vi "查询-累积剂量记录.vi"() -> ()   [LabVIEW 2017]
uses:
  <vilib>/addons/database/Connection.llb/Conn ObjectReference.ctl
  <vilib>/Utility/inputDevices.llb/mouseAcquire.vi
  <vilib>/addons/database/NI_Database_API.lvlib
panel:
  out "信号-导出数据":bool=TRUE
  in  "停止？":bool=TRUE
  in  "提示-条件区域[]":string[](array[string])
  in  "提示-数据列表[]":string[](array[string])
  in  "提示-设备列表[]":string[](array[string])
  out "信号-重连DB":bool=TRUE
  in  "device ID":refnum<k1> caption="设备ID"
  out "信号-刷新功能管理表":bool=TRUE
  out "最小记录时间":i32[](array[numeric])
  out "DB 引用":T1
  out "累积功能管理":enum16{"设备列表"}(ring)
  out "提示-设备列表":string
  in  "全选-设备":bool
  in  "查询条件":T2
  in  "设备累积管理":i32[](listbox)
  out "累积剂量查询":enum16{"累积剂量查询"}(ring)
  out "提示-数据列表":string
  in  "记录类型":enum16{"全部记录", "报警记录"}(ring)
  in  "全选-记录":bool
  in  "记录列表":i32[](listbox)
  out "查询条件":enum16{"查询条件"}(ring)
  out "提示-条件区域":string
  out "查询状态":string
  out "选中状态":string
  out "起始时间":enum16{"起始时间"}(ring)
  in  "从今天":bool
  in  "起始年":u16(ring) items=["2017年"=2017]
  in  "起始月":u16(ring) items=["1月"=1, "2月"=2, "3月"=3, "4月"=4, "5月"=5, "6月"=6, "7月"=7, "8月"=8, "9月"=9, "10月"=10, "11月"=11, "12月"=12]
  in  "起始日":u16(ring) items=["1日"=1, "2日"=2, "3日"=3, "4日"=4, "5日"=5, "6日"=6, "7日"=7, "8日"=8, "9日"=9, "10日"=10, "11日"=11, "12日"=12, "13日"=13, "14日"=14, "15日"=15, "16日"=16, "17日"=17, "18日"=18, "19日"=19, "20日"=20, "21日"=21, "22日"=22, "23日"=23, "24日"=24, "25日"=25, "26日"=26, "27日"=27, "28日"=28, "29日"=29, "30日"=30, "31日"=31]
  out "截止时间":enum16{"截止时间"}(ring)
  in  "到今天":bool
  in  "截止年":u16(ring) items=["2017年"=2017]
  in  "截止月":u16(ring) items=["1月"=1, "2月"=2, "3月"=3, "4月"=4, "5月"=5, "6月"=6, "7月"=7, "8月"=8, "9月"=9, "10月"=10, "11月"=11, "12月"=12]
  in  "截止日":u16(ring) items=["1日"=1, "2日"=2, "3日"=3, "4日"=4, "5日"=5, "6日"=6, "7日"=7, "8日"=8, "9日"=9, "10日"=10, "11日"=11, "12日"=12, "13日"=13, "14日"=14, "15日"=15, "16日"=16, "17日"=17, "18日"=18, "19日"=19, "20日"=20, "21日"=21, "22日"=22, "23日"=23, "24日"=24, "25日"=25, "26日"=26, "27日"=27, "28日"=28, "29日"=29, "30日"=30, "31日"=31]
  in  "导出数据":bool
  in  "查询今日":bool
  in  "查看导出目录":bool
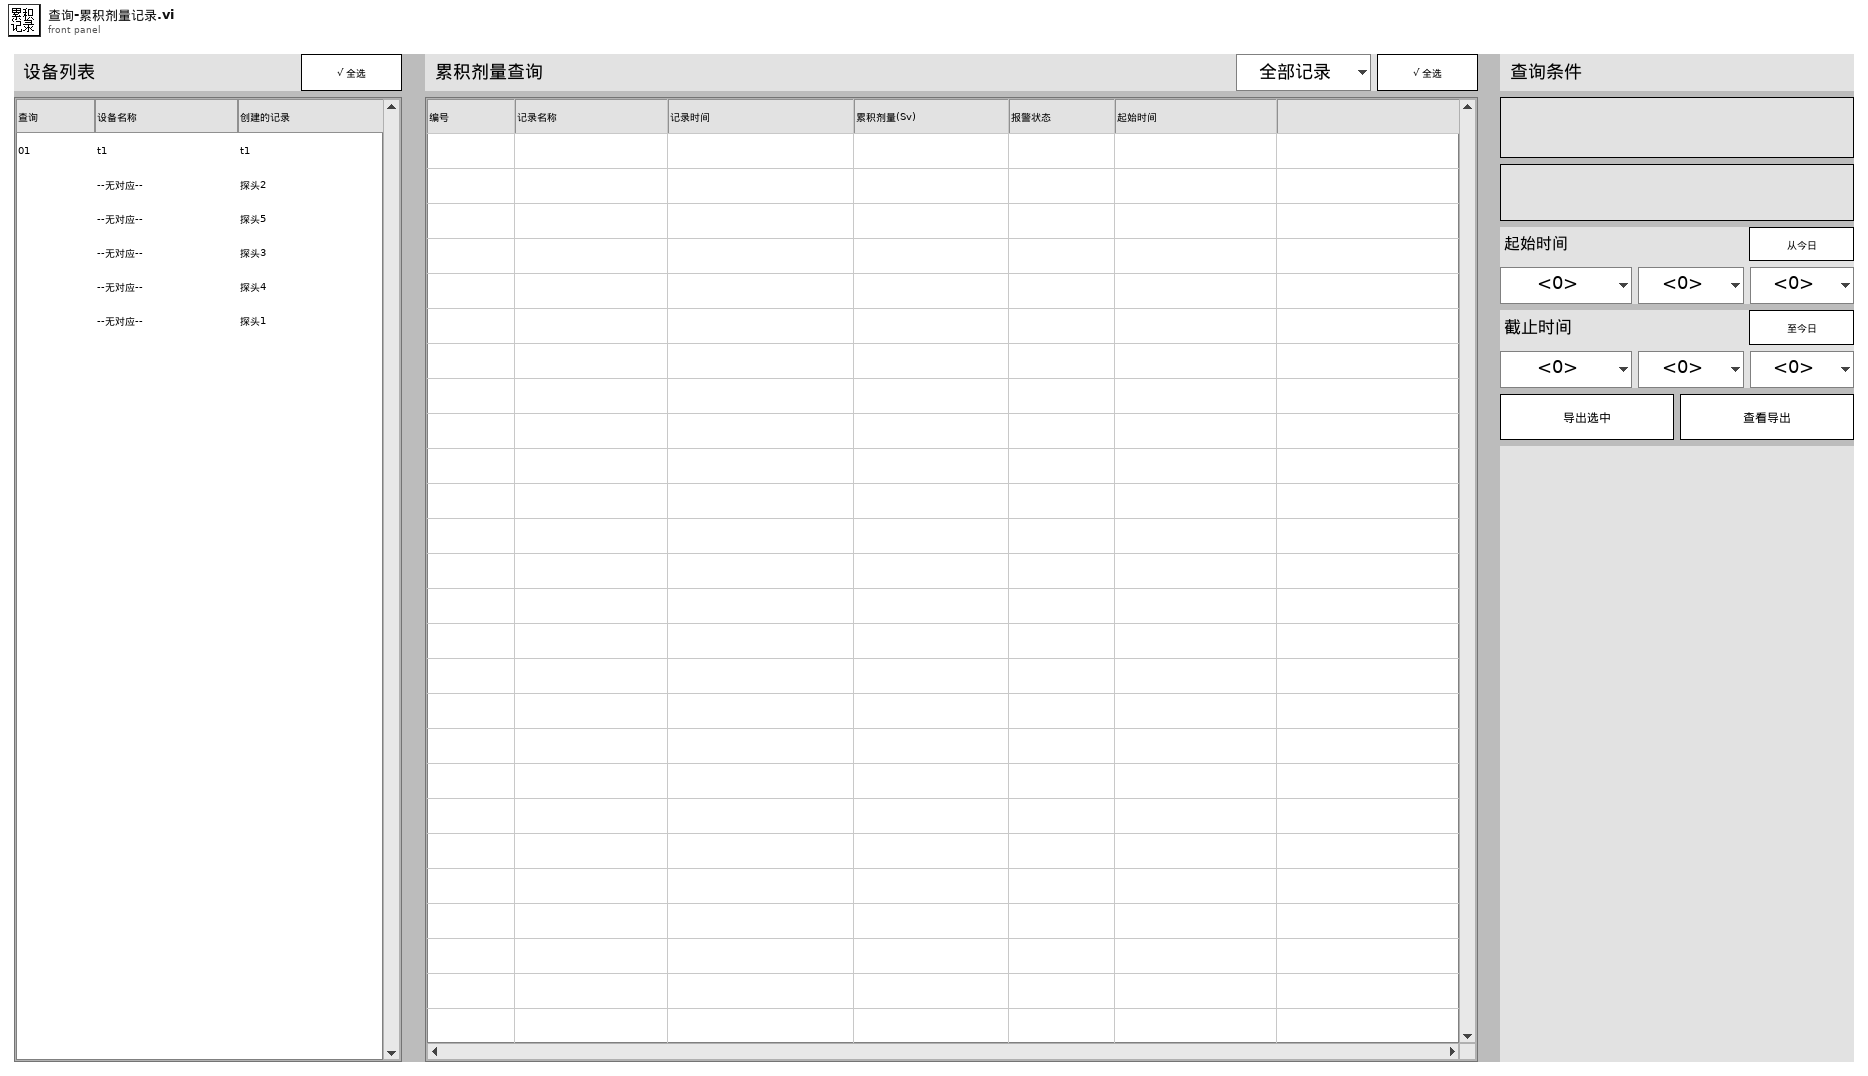
[diagram p1: front panel]
types:
  T1 = typedef "NI_Database_API.lvlib/Conn ObjectReference.ctl" = refnum<k1>
  T2 = cluster{"表名":string[], "起始时间":string, "截止时间":string, "优先排序":enum16{"表名优先", "记录时间优先"}, "排序方向":enum16{"升序", "降序"}, "记录类型":enum16{"全部记录", "报警记录"}}
  T3 = cluster{"设备名称":string, "启用累积？":bool, "起始时间":timestamp, "累积剂量":dbl, "累积报警阈值":dbl}
  T4 = typedef "LVDateTimeRec.ctl" = cluster{"秒数的小数部分":dbl, "秒":i32, "分":i32, "时":i32, "日":i32, "月":i32, "年":i32, "天数（周）":i32, "天数（年）":i32, "DST":i32}
  T5 = typedef "LVPoint32TypeDef.ctl" = cluster{"Horizontal":i32, "Vertical":i32}
  T6 = cluster{"button 1":bool, "button 2":bool, "button 3":bool, "button 4":bool}
  T7 = typedef "LVRowAndColumnTypeDef.ctl" = cluster{"Row":i32, "Column":i32}
  T8 = cluster{"设备名称":string, "启用累积？":bool, "起始时间":timestamp, "累积剂量":dbl, "累积报警阈值":dbl}[]
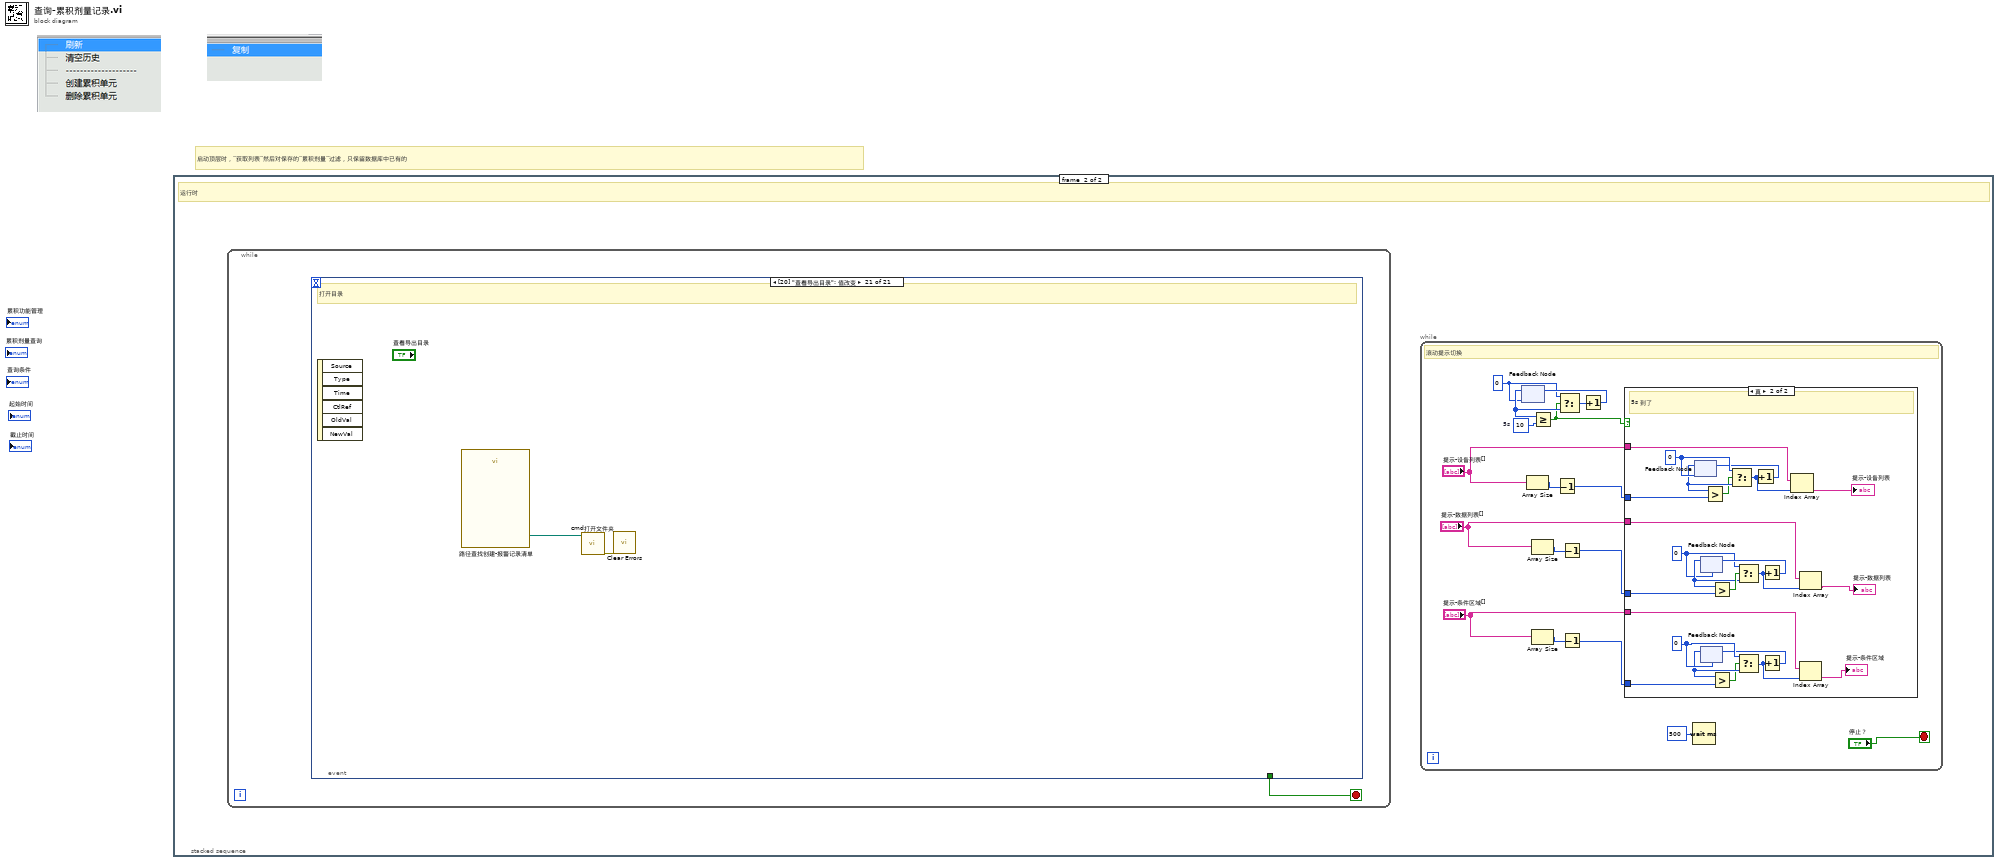
[diagram p0: block diagram]
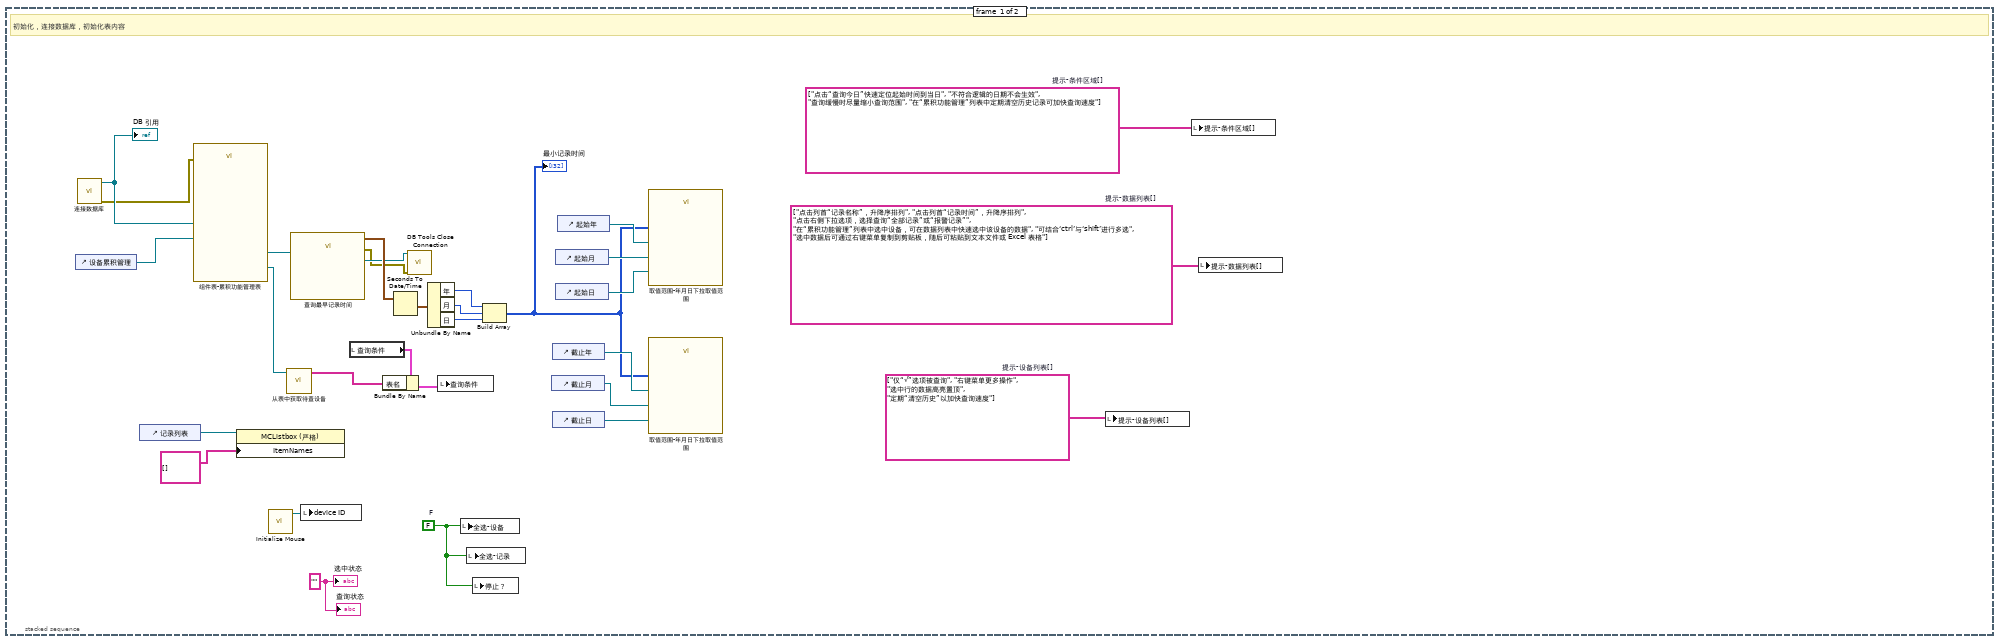
[diagram p2: hidden frame]
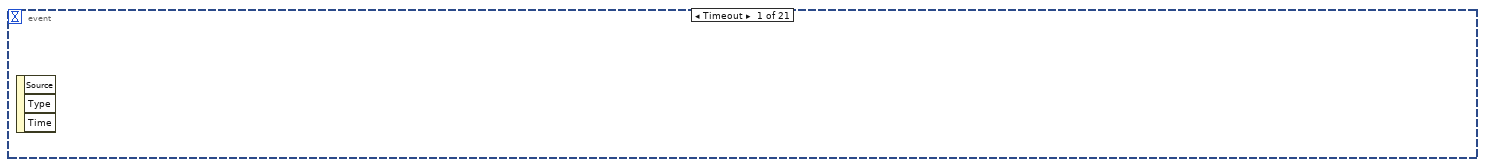
[diagram p4: hidden frame]
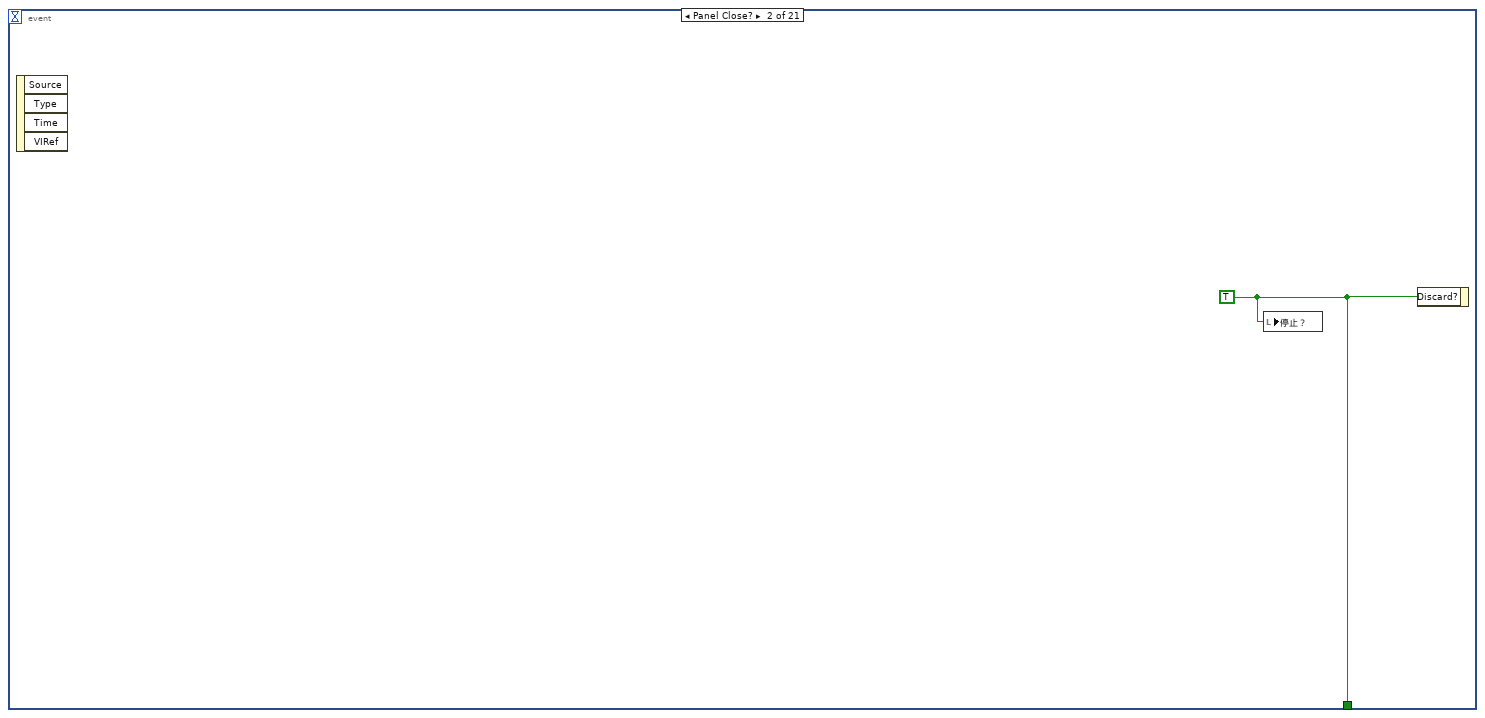
[diagram p5: hidden frame]
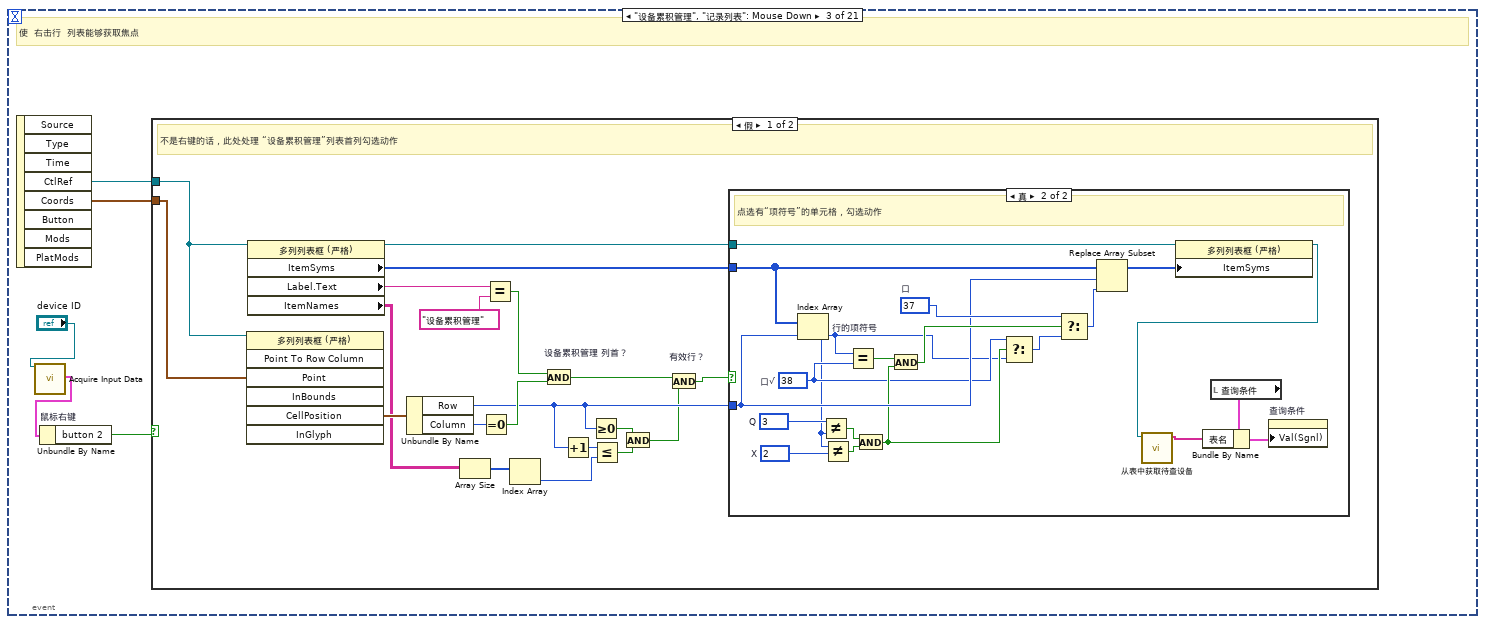
[diagram p6: hidden frame]
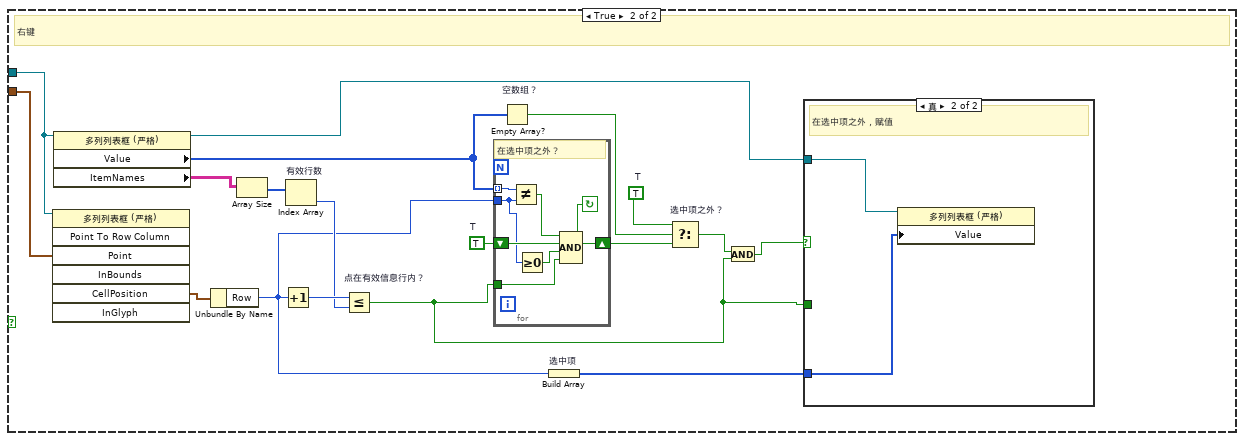
[diagram p8: hidden frame]
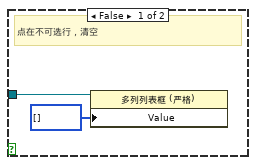
[diagram p10: hidden frame]
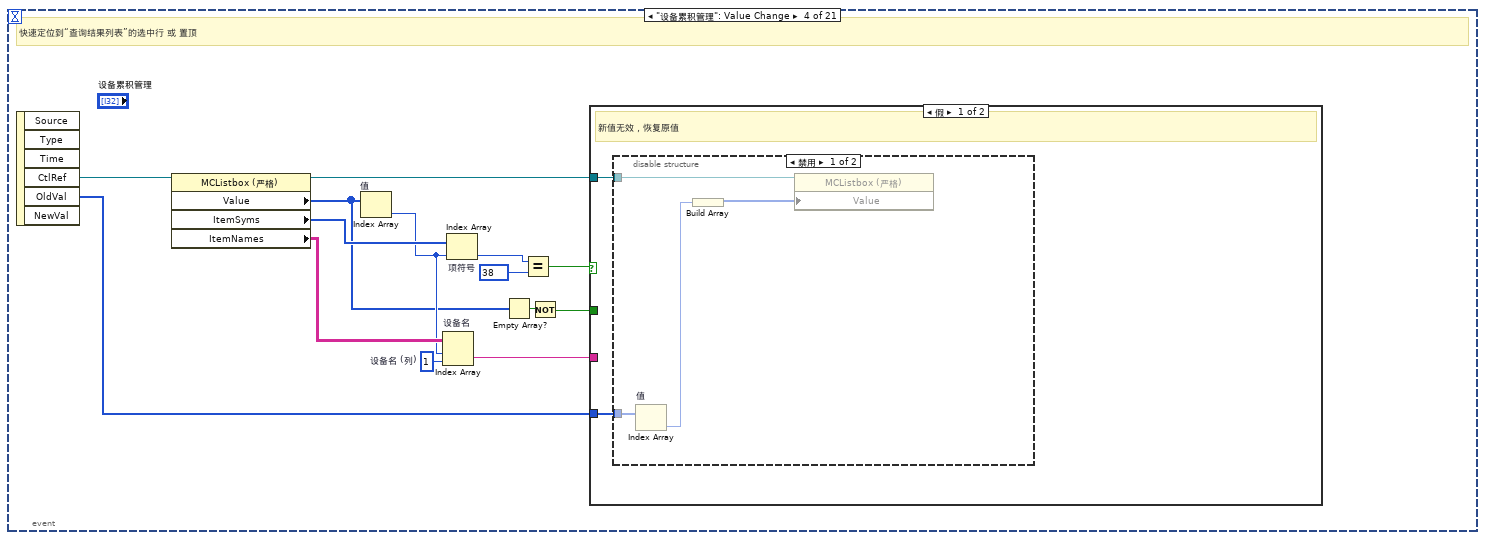
[diagram p11: hidden frame]
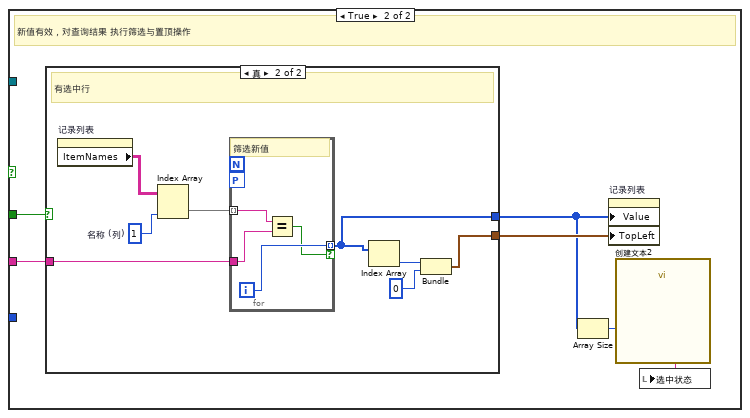
[diagram p13: hidden frame]
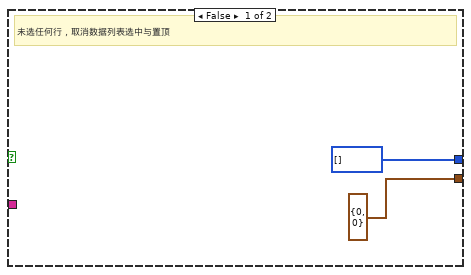
[diagram p14: hidden frame]
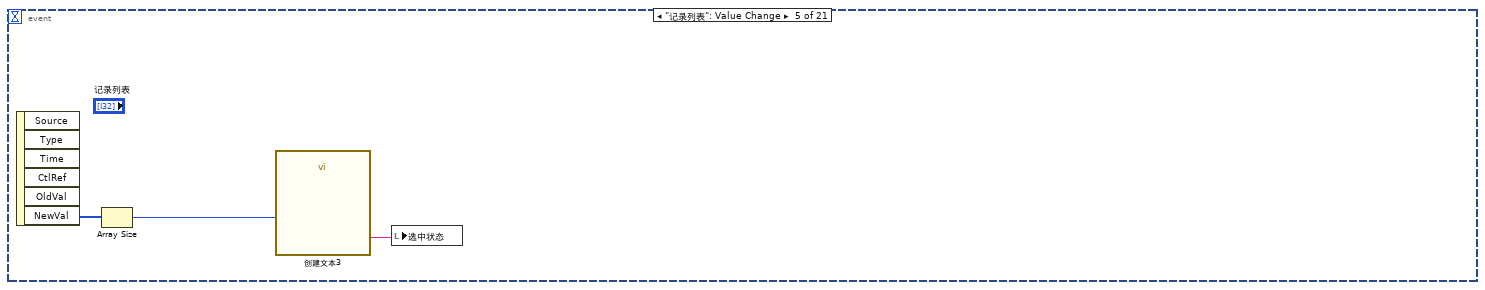
[diagram p15: hidden frame]
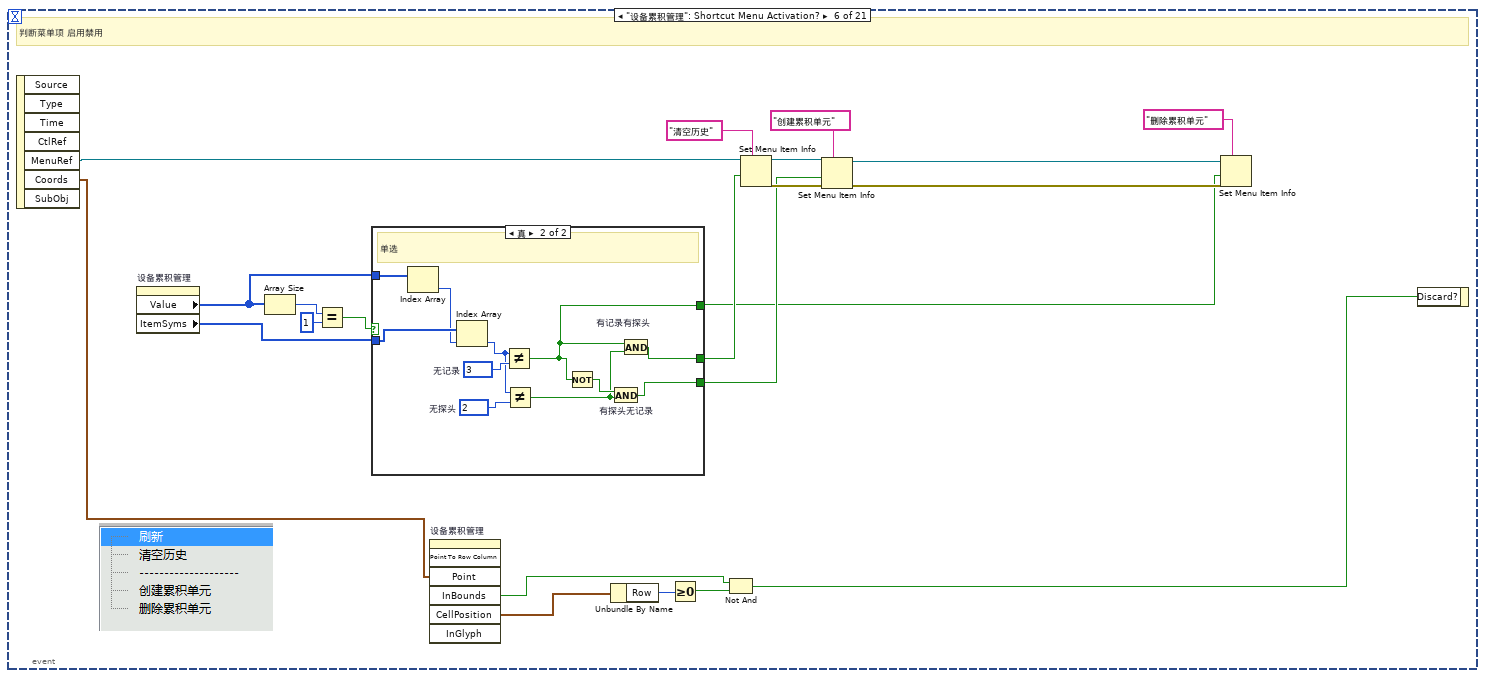
[diagram p16: hidden frame]
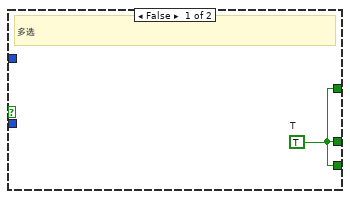
[diagram p17: hidden frame]
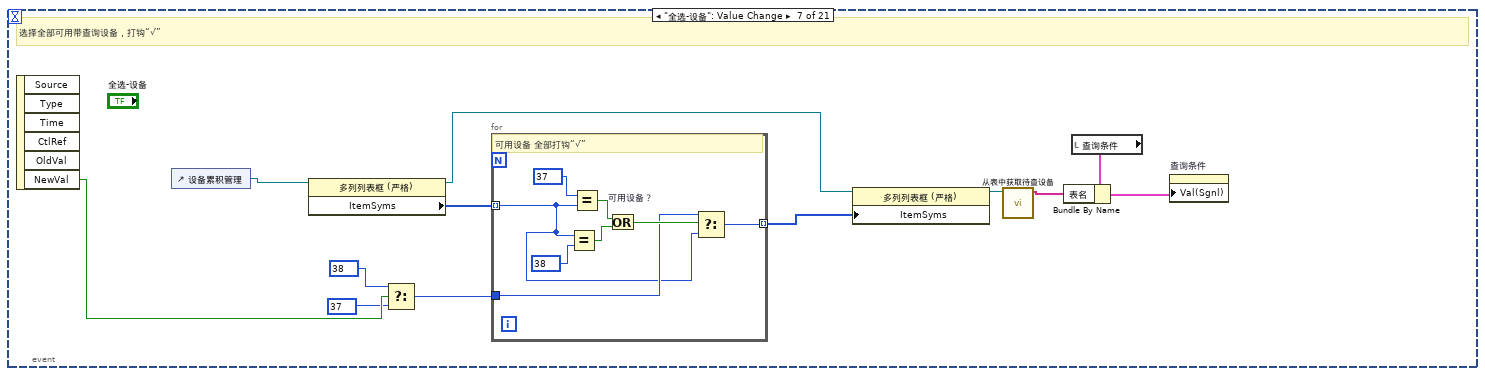
[diagram p18: hidden frame]
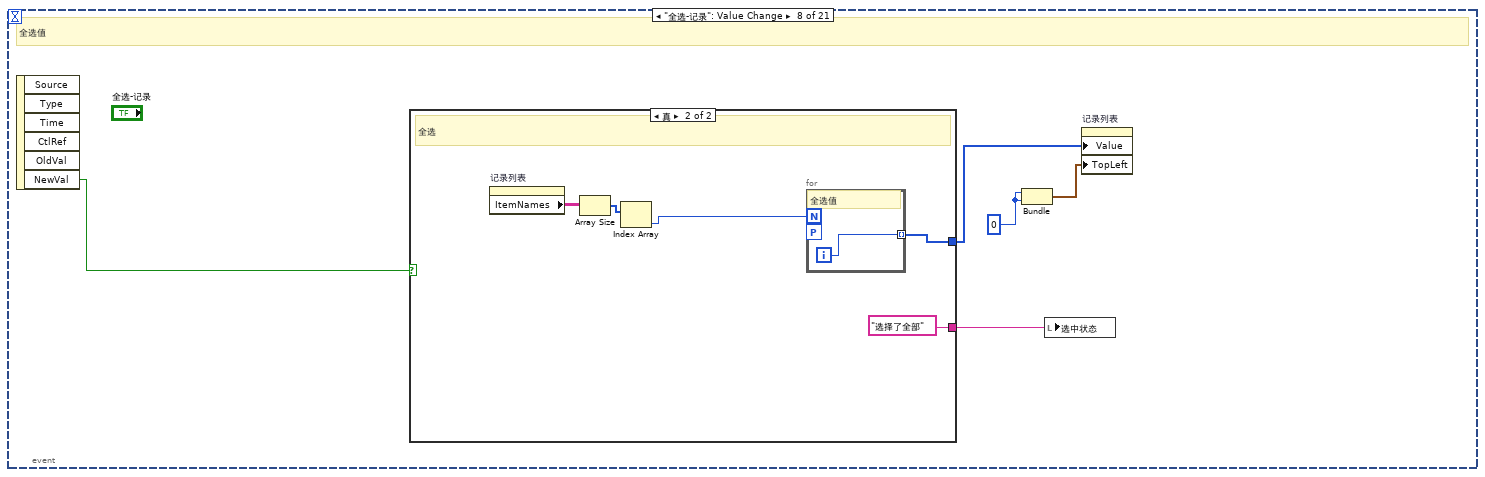
[diagram p19: hidden frame]
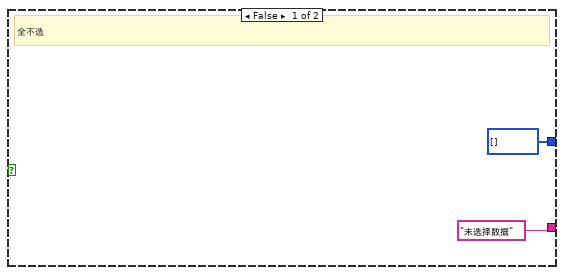
[diagram p20: hidden frame]
diagram:
  # "启动顶层时，“获取列表”然后对保存的“累积剂量”过滤，只保留数据库中已有的"
  n1 = stacked-sequence {
    frame #0 {
      w9 = string[] ["点击“查询今日”快速定位起始时间到当日", "不符合逻辑的日期不会生效", "查询缓慢时尽量缩小查询范围", "在“累积功能管理”列表中定期清空历史记录可加快查询速度"]  # 提示-条件区域[]
      w8 = string[] ["点击列首“记录名称”，升降序排列", "点击列首“记录时间”，升降序排列", "点击右侧下拉选项，选择查询“全部记录”或“报警记录”", "在“累积功能管理”列表中选中设备，可在数据列表中快速选中该设备的数据", "可结合‘ctrl’与‘shift’进行多选", "选中数据后可通过右键菜单复制到剪贴板，随后可粘贴到文本文件或 Excel 表格"]  # 提示-数据列表[]
      w10 = "" ("选中状态")
      w7 = string[] ["仅“√”选项被查询", "右键菜单更多操作", "选中行的数据高亮置顶", "定期“清空历史”以加快查询速度"]  # 提示-设备列表[]
      w6 = FALSE  # F
      # "初始化，连接数据库，初始化表内容"
      n2 = control-ref of="设备累积管理"() -> (w30:refnum<vi>)
      n3 = call "连接数据库.vi"() -> ("error out"=w3:errorcluster, "connection reference"=w16:T1)  [unwired: 10 in]
      "DB 引用" <- w16
      n4 = control-ref of="记录列表"() -> (w5:refnum<vi>)
      n5 = call "组件表-累积功能管理表.vi"("引用-累积功能管理列表"=w30, "error in (no error)"=w3, "DB 引用"=w16) -> ("数据库连接引用 o"=w29:T1, "引用-累积功能管理表 o"=w14:refnum<vi>)  [unwired: 6 in, 1 out]
      n6 = property class="MCListbox (严格)"(reference=w5, "ItemNames"=string[][] [] ("项名")) -> ()  [unwired: 1 in, 2 out]
      n7 = call <vilib>:"Initialize Mouse.vi"() -> ("device ID"=w15:refnum<k1>)  [unwired: 10 in, 1 out]
      n8 = call "从表中获取待查设备.vi"("引用-设备累积管理 i"=w14) -> ("选中的查询设备"=w12:string[])  [unwired: 10 in]
      n9 = call "查询最早记录时间.vi"("DB 引用"=w29) -> ("error out"=w1:errorcluster, "最小记录时间"=w22:timestamp, "数据库连接引用out"=w2:T1)  [unwired: 8 in]
      n10 = local write "device ID"(w15) -> ()
      n11 = local read "查询条件"() -> (w13:T2)
      n12 = Bundle By Name(cluster=w13, "表名"=w12) -> (w11:T2)
      n13 = Seconds To Date/Time(time stamp (now)=w22) -> (date time rec=w21:T4)  [unwired: 1 in]
      n14 = call <vilib>:"DB Tools Close Connection.vi"("error in (no error)"=w1, "connection reference"=w2) -> ()  [unwired: 5 in, 1 out]
      n15 = Unbundle By Name(w21) -> ("年"=w20:i32, "月"=w19:i32, "日"=w18:i32)
      n16 = local write "查询条件"(w11) -> ()
      n17 = local write "全选-设备"(w6) -> ()
      n18 = local write "全选-记录"(w6) -> ()
      n19 = local write "停止？"(w6) -> ()
      n20 = Build Array(w20, w19, w18) -> (w17:i32[])
      "最小记录时间" <- w17
      n21 = control-ref of="截止月"() -> (w24:refnum<vi>)
      n22 = control-ref of="截止年"() -> (w25:refnum<vi>)
      n23 = control-ref of="截止日"() -> (w23:refnum<vi>)
      n24 = control-ref of="起始月"() -> (w27:refnum<vi>)
      n25 = control-ref of="起始日"() -> (w26:refnum<vi>)
      n26 = control-ref of="起始年"() -> (w28:refnum<vi>)
      n27 = call "取值范围-年月日下拉取值范围.vi"("最小日期"=w17, "日"=w26, "月"=w27, "年"=w28) -> ()  [unwired: 7 in, 1 out]
      n28 = call "取值范围-年月日下拉取值范围.vi"("最小日期"=w17, "日"=w23, "月"=w24, "年"=w25) -> ()  [unwired: 7 in, 1 out]
      n29 = local write "提示-设备列表[]"(w7) -> ()
      n30 = local write "提示-条件区域[]"(w9) -> ()
      n31 = local write "提示-数据列表[]"(w8) -> ()
      "查询状态" <- w10
      "选中状态" <- w10
    }
    frame #1 {
      # "运行时"
      n32 = while {
        stop <- w72 stop-if-true
        n33 = event shown="[20] \"查看导出目录\": 值改变" {
          selector: _ -> [_ _ _ _ _ _ _ _ _ _ _ _ _ _ _ _ _ _ _ _ _]
          dyn-events: _ -> [_ _ _ _ _ _ _ _ _ _ _ _ _ _ _ _ _ _ _ _ _]
          timeout: _ -> [_ _ _ _ _ _ _ _ _ _ _ _ _ _ _ _ _ _ _ _ _]
          tunnel: [_ w73 _ _ _ _ _ _ _ _ _ _ _ _ _ _ _ _ _ _ _] -> w72
          event Timeout {
            n34 = event-data() -> ()  [unwired: 1 in, 3 out]
          }
          event Panel Close? {
            w73 = TRUE ("放弃？")
            n35 = event-data() -> ()  [unwired: 1 in, 4 out]
            n36 = local write "停止？"(w73) -> ()
            n37 = event-data("Discard?"=w73) -> ()  [unwired: 1 in, 1 out]
          }
          event "设备累积管理", "记录列表": Mouse Down {
            # "使  右击行  列表能够获取焦点"
            n38 = event-data() -> ("CtlRef"=w75:refnum<vi>, "Coords"=w76:T5)  [unwired: 1 in, 6 out]
            n39 = call-poly <vilib>:"Acquire Input Data.vi"("device ID"="device ID") -> ("button info"=w78:T6)  [unwired: 15 in, 3 out]
            n40 = Unbundle By Name "鼠标右键"(w78) -> ("button 2"=w74:bool)
            n41 = case shown="假" w74 {
              tunnel: w76 -> [w98 w136]
              tunnel: w75 -> [w97 w135]
              frame False {
                # "不是右键的话，此处处理 “设备累积管理”列表首列勾选动作"
                n42 = invoke class="多列列表框 (严格)" method="Point To Row Column"(reference=w97, "Point"=w98) -> ("CellPosition"=w92:T7)  [unwired: 5 in, 6 out]
                n43 = property class="多列列表框 (严格)"(reference=w97) -> (reference out=w89:refnum<vi>, "ItemSyms"=w88:i32[], "Label.Text"=w93:string, "ItemNames"=w86:string[][])  [unwired: 1 in, 1 out]
                n44 = Unbundle By Name(w92) -> ("Row"=w81:i32, "Column"=w91:i32)
                n45 = Array Size(array=w86) -> (size(s)=w87:i32[])
                n46 = Equal To 0?(x=w91) -> (x = 0?=w95:bool)
                n47 = Equal?(x=w93, y="设备累积管理") -> (x = y?=w94:bool)
                n48 = Index Array(array=w87) -> (element=w84:i32)  [unwired: 1 in]
                n49 = And "设备累积管理 列首？"(x=w94, y=w95) -> (x .and. y?=w90:bool)
                n50 = Increment(x=w81) -> (x+1=w85:i32)
                n51 = Greater Or Equal To 0?(x=w81) -> (x >= 0?=w82:bool)
                n52 = Less Or Equal?(x=w85, y=w84) -> (x <= y?=w83:bool)
                n53 = And(x=w82, y=w83) -> (x .and. y?=w79:bool)
                n54 = And "有效行？"(x=w90, y=w79) -> (x .and. y?=w80:bool)
                n55 = case shown="真" w80 {
                  tunnel: w81 -> [_ w103]
                  tunnel: w89 -> [_ w118]
                  tunnel: w88 -> [_ w115]
                  frame False {
                  }
                  frame True {
                    w107 = 2  # X
                    w108 = 3  # Q
                    w101 = 38  # 口√
                    w116 = 37  # 口
                    # "点选有“项符号”的单元格，勾选动作"
                    n56 = Index Array "行的项符号"(array=w115, index=w103) -> (element=w100:i32)
                    n57 = Not Equal?(x=w108, y=w100) -> (x != y?=w105:bool)
                    n58 = Not Equal?(x=w100, y=w107) -> (x != y?=w106:bool)
                    n59 = Equal?(x=w100, y=w101) -> (x = y?=w117:bool)
                    n60 = And(x=w105, y=w106) -> (x .and. y?=w102:bool)
                    n61 = And(x=w117, y=w102) -> (x .and. y?=w104:bool)
                    n62 = Select(t=w101, s=w102, f=w100) -> (s? t:f=w99:i32)
                    n63 = Select(t=w116, s=w104, f=w99) -> (s? t:f=w114:i32)
                    n64 = Replace Array Subset(array=w115, new element=w114, index=w103) -> (w113:i32[])
                    n65 = property class="多列列表框 (严格)"(reference=w118, "ItemSyms"=w113) -> (reference out=w112:refnum<vi>)  [unwired: 1 in, 1 out]
                    n66 = call "从表中获取待查设备.vi"("引用-设备累积管理 i"=w112) -> ("选中的查询设备"=w110:string[])  [unwired: 10 in]
                    n67 = local read "查询条件"() -> (w111:T2)
                    n68 = Bundle By Name(cluster=w111, "表名"=w110) -> (w109:T2)
                    n69 = property on="查询条件" class="Clust (严格)"("Val(Sgnl)"=w109) -> ()  [unwired: 2 in, 2 out]
                  }
                }
              }
              frame True {
                w127 = TRUE  # T
                w128 = TRUE  # T
                # "右键"
                n70 = invoke class="多列列表框 (严格)" method="Point To Row Column"(reference=w135, "Point"=w136) -> ("CellPosition"=w132:T7)  [unwired: 5 in, 6 out]
                n71 = property class="多列列表框 (严格)"(reference=w135) -> (reference out=w121:refnum<vi>, "Value"=w129:i32[], "ItemNames"=w134:string[][])  [unwired: 1 in, 1 out]
                n72 = Unbundle By Name(w132) -> ("Row"=w123:i32)
                n73 = Array Size(array=w134) -> (size(s)=w133:i32[])
                n74 = Increment(x=w123) -> (x+1=w131:i32)
                n75 = Index Array "有效行数"(array=w133) -> (element=w130:i32)  [unwired: 1 in]
                n76 = Less Or Equal? "点在有效信息行内？"(x=w131, y=w130) -> (x <= y?=w119:bool)
                n77 = for {
                  tunnel: w129 -> [w149] mode=indexing
                  shift-right: [w146] -> w125
                  shift-left: w128 -> [w147]
                  tunnel: w123 -> [w145]
                  tunnel: w119 -> [w143]
                  stop <- w146 continue-if-true
                  # "在选中项之外？"
                  n78 = Not Equal?(x=w149, y=w145) -> (x != y?=w148:bool)
                  n79 = Greater Or Equal To 0?(x=w145) -> (x >= 0?=w144:bool)
                  n80 = Compound Arithmetic op=AND(w148, w147, w144, w143) -> (w146:bool)
                }
                n81 = Empty Array? "空数组？"(array=w129) -> (empty?=w126:bool)
                n82 = Build Array "选中项"(w123) -> (w122:i32[])
                n83 = Select "选中项之外？"(t=w127, s=w126, f=w125) -> (s? t:f=w124:bool)
                n84 = And(x=w124, y=w119) -> (x .and. y?=w120:bool)
                n85 = case shown="真" w120 {
                  tunnel: w122 -> [_ w141]
                  tunnel: w121 -> [w137 w142]
                  tunnel: w119 -> [w138 _]
                  frame False {
                    # "在选中项之中，不赋值"
                    n86 = case shown="真" w138 {
                      tunnel: w137 -> [w140 _]
                      frame False {
                        # "点在不可选行，清空"
                        n87 = property class="多列列表框 (严格)"(reference=w140, "Value"=i32[] [] ("值")) -> ()  [unwired: 1 in, 2 out]
                      }
                      frame True {
                      }
                    }
                  }
                  frame True {
                    # "在选中项之外，赋值"
                    n88 = property class="多列列表框 (严格)"(reference=w142, "Value"=w141) -> ()  [unwired: 1 in, 2 out]
                  }
                }
              }
            }
          }
          event "设备累积管理": Value Change {
            w161 = 1  # 设备名 (列)
            # "快速定位到“查询结果列表”的选中行 或 置顶"
            n89 = event-data() -> ("CtlRef"=w163:refnum<vi>, "OldVal"=w156:i32[])  [unwired: 1 in, 4 out]
            n90 = property class="MCListbox (严格)"(reference=w163) -> (reference out=w155:refnum<vi>, "Value"=w152:i32[], "ItemSyms"=w160:i32[], "ItemNames"=w162:string[][])  [unwired: 1 in, 1 out]
            n91 = Index Array "值"(array=w152) -> (element=w153:i32)  [unwired: 1 in]
            n92 = Index Array "设备名"(array=w162, index (row)=w153, index (col)=w161) -> (element=w154:string)
            n93 = Index Array "项符号"(array=w160, index=w153) -> (element=w159:i32)
            n94 = Empty Array?(array=w152) -> (empty?=w151:bool)
            n95 = Equal?(x=w159, y=38) -> (x = y?=w157:bool)
            n96 = Not(x=w151) -> (.not. x?=w150:bool)
            n97 = case shown="假" w157 {
              tunnel: w156 -> [w164 _]
              tunnel: w155 -> [w165 _]
              tunnel: w154 -> [_ w175]
              tunnel: w150 -> [_ w174]
              frame False {
                # "新值无效，恢复原值"
                n98 = disable-structure shown="禁用" {
                  disable-tunnel: w165 -> [w167 _]
                  disable-tunnel: w164 -> [w166 _]
                  frame Disabled {
                    n99 = Index Array "值"(array=w166) -> (element=w169:i32)  [unwired: 1 in]
                    n100 = Build Array(w169) -> (w168:i32[])
                    n101 = property class="MCListbox (严格)"(reference=w167, "Value"=w168) -> ()  [unwired: 1 in, 2 out]
                  }
                  frame Enabled {
                  }
                }
              }
              frame True {
                # "新值有效，对查询结果 执行筛选与置顶操作"
                n102 = case shown="真" w174 {
                  tunnel: w175 -> [_ w182]
                  tunnel: [i32[] [] w179] -> w172
                  tunnel: [cluster{i32, i32} {0, 0} w178] -> w173
                  frame False {
                    # "未选任何行，取消数据列表选中与置顶"
                  }
                  frame True {
                    w184 = 1  # 名称 (列)
                    # "有选中行"
                    n103 = property on="记录列表" class="MCListbox (严格)"() -> ("ItemNames"=w185:string[][])  [unwired: 2 in, 2 out]
                    n104 = Index Array(array=w185, index (col)=w184) -> (element=w183:string[])  [unwired: 1 in]
                    n105 = for {
                      workers-P: _ -> [_]
                      tunnel: w183 -> [w189] mode=indexing
                      tunnel: w182 -> [w188]
                      tunnel: [w187] -> w179 mode=indexing if=w186
                      i -> [w187]
                      # "筛选新值"
                      n106 = Equal?(x=w189, y=w188) -> (x = y?=w186:bool)
                    }
                    n107 = Index Array(array=w179) -> (element=w181:i32)  [unwired: 1 in]
                    n108 = Bundle(w181, 0) -> (w178:cluster{i32, i32})  [unwired: 1 in]
                  }
                }
                n109 = Array Size(array=w172) -> (size(s)=w171:i32)
                n110 = property on="记录列表" class="MCListbox (严格)"("Value"=w172, "TopLeft"=w173) -> ()  [unwired: 2 in, 2 out]
                n111 = call "创建文本2"("选中条数"=w171) -> ("Result"=w170:string)  [unwired: 13 in, 1 out]
                n112 = local write "选中状态"(w170) -> ()
              }
            }
          }
          event "记录列表": Value Change {
            n113 = event-data() -> ("NewVal"=w192:i32[])  [unwired: 1 in, 5 out]
            n114 = Array Size(array=w192) -> (size(s)=w191:i32)
            n115 = call "创建文本3"("选中条数"=w191) -> ("Result"=w190:string)  [unwired: 13 in, 1 out]
            n116 = local write "选中状态"(w190) -> ()
          }
          event "设备累积管理": Shortcut Menu Activation? {
            # "判断菜单项 启用禁用"
            n117 = event-data() -> ("MenuRef"=w207:refnum<k9>, "Coords"=w198:T5)  [unwired: 1 in, 5 out]
            n118 = property on="设备累积管理" class="MCListbox (严格)"() -> ("Value"=w206:i32[], "ItemSyms"=w205:i32[])  [unwired: 2 in, 2 out]
            n119 = Array Size(array=w206) -> (size(s)=w214:i32)
            n120 = Equal?(x=w214, y=1) -> (x = y?=w212:bool)
            n121 = case shown="真" w212 {
              tunnel: w206 -> [_ w226]
              tunnel: w205 -> [_ w225]
              tunnel: [w215 w222] -> w201
              tunnel: [w215 w219] -> w200
              tunnel: [w215 w216] -> w199
              frame False {
                w215 = TRUE  # T
                # "多选"
              }
              frame True {
                w220 = 2  # 无探头
                w223 = 3  # 无记录
                # "单选"
                n122 = Index Array(array=w226) -> (element=w224:i32)  [unwired: 1 in]
                n123 = Index Array(array=w225, index=w224) -> (element=w221:i32)
                n124 = Not Equal? ("可用？")(x=w221, y=w223) -> (x != y?=w216:bool)
                n125 = Not Equal? ("可用？")(x=w221, y=w220) -> (x != y?=w217:bool)
                n126 = Not(x=w216) -> (.not. x?=w218:bool)
                n127 = And "有探头无记录"(x=w218, y=w217) -> (x .and. y?=w219:bool)
                n128 = And "有记录有探头"(x=w216, y=w217) -> (x .and. y?=w222:bool)
              }
            }
            n129 = invoke on="设备累积管理" class="多列列表框 (严格)" method="Point To Row Column"("Point"=w198) -> ("InBounds"=w194:bool, "CellPosition"=w197:T7)  [unwired: 6 in, 5 out]
            n130 = Unbundle By Name(w197) -> ("Row"=w196:i32)
            n131 = Greater Or Equal To 0?(x=w196) -> (x >= 0?=w195:bool)
            n132 = Not And(1:w195, 2:w194) -> (0:w193:bool)
            n133 = Set Menu Item Info(7:"清空历史", 9:w201, 11:w207) -> (0:w209:errorcluster, 3:w208:refnum<k9>)  [unwired: 4 in]
            n134 = Set Menu Item Info(7:"创建累积单元", 8:w209, 9:w200, 11:w208) -> (0:w210:errorcluster, 3:w211:refnum<k9>)  [unwired: 3 in]
            n135 = Set Menu Item Info(7:"删除累积单元", 8:w210, 9:w199, 11:w211) -> ()  [unwired: 3 in, 2 out]
            n136 = event-data("Discard?"=w193) -> ()  [unwired: 1 in, 1 out]
          }
          event "全选-设备": Value Change {
            # "选择全部可用带查询设备，打钩“√”"
            n137 = event-data() -> ("NewVal"=w230:bool)  [unwired: 1 in, 5 out]
            n138 = control-ref of="设备累积管理"() -> (w233:refnum<vi>)
            n139 = property on="属性节点" class="多列列表框 (严格)"(reference=w233) -> (reference out=w232:refnum<vi>, "ItemSyms"=w238:i32[])  [unwired: 1 in, 1 out]
            n140 = Select(t=38, s=w230, f=37) -> (s? t:f=w227:i32)
            n141 = for {
              tunnel: w238 -> [w240] mode=indexing
              tunnel: [w239] -> w237 mode=indexing
              tunnel: w227 -> [w241]
              # "可用设备 全部打钩“√”"
              n142 = Equal?(x=w240, y=38) -> (x = y?=w246:bool)
              n143 = Equal?(x=37, y=w240) -> (x = y?=w245:bool)
              n144 = Or "可用设备？"(x=w245, y=w246) -> (x .or. y?=w242:bool)
              n145 = Select(t=w241, s=w242, f=w240) -> (s? t:f=w239:i32)
            }
            n146 = property on="属性节点" class="多列列表框 (严格)"(reference=w232, "ItemSyms"=w237) -> (reference out=w231:refnum<vi>)  [unwired: 1 in, 1 out]
            n147 = call "从表中获取待查设备.vi"("引用-设备累积管理 i"=w231) -> ("选中的查询设备"=w235:string[])  [unwired: 10 in]
            n148 = local read "查询条件"() -> (w236:T2)
            n149 = Bundle By Name(cluster=w236, "表名"=w235) -> (w234:T2)
            n150 = property on="查询条件" class="Clust (严格)"("Val(Sgnl)"=w234) -> ()  [unwired: 2 in, 2 out]
          }
          event "全选-记录": Value Change {
            w250 = 0
            # "全选值"
            n151 = event-data() -> ("NewVal"=w251:bool)  [unwired: 1 in, 5 out]
            n152 = case shown="真" w251 {
              tunnel: [i32[] [] w258] -> w248
              tunnel: ["未选择数据" ("选中状态") "选择了全部" ("选中状态")] -> w247
              frame False {
                # "全不选"
              }
              frame True {
                # "全选"
                n153 = property on="记录列表" class="MCListbox (严格)"() -> ("ItemNames"=w256:string[][])  [unwired: 2 in, 2 out]
                n154 = Array Size(array=w256) -> (size(s)=w257:i32[])
                n155 = Index Array(array=w257) -> (element=w255:i32)  [unwired: 1 in]
                n156 = for {
                  N: w255 -> [_]
                  workers-P: _ -> [_]
                  tunnel: [w259] -> w258 mode=indexing
                  i -> [w259]
                  # "全选值"
                }
              }
            }
            n157 = Bundle(w250, w250) -> (w249:cluster{i32, i32})  [unwired: 1 in]
            n158 = local write "选中状态"(w247) -> ()
            n159 = property on="记录列表" class="MCListbox (严格)"("Value"=w248, "TopLeft"=w249) -> ()  [unwired: 2 in, 2 out]
          }
          event "记录类型": Value Change {
            n160 = event-data() -> ()  [unwired: 1 in, 6 out]
            n161 = local read "查询条件"() -> (w262:T2)
            n162 = Bundle By Name(cluster=w262, "记录类型"="记录类型") -> (w261:T2)
            n163 = property on="查询条件" class="Clust (严格)"("Val(Sgnl)"=w261) -> ()  [unwired: 2 in, 2 out]
          }
          event "设备累积管理": Shortcut Menu Selection (User) {
            # "执行菜单事件"
            n164 = event-data() -> ("CtlRef"=w267:refnum<vi>, "ItemTag"=w268:string)  [unwired: 1 in, 6 out]
            n165 = global read "全局变量-35点监测.vi" "引用-累积剂量[]"() -> (w266:refnum<vi>)
            n166 = call "连接数据库.vi"() -> ("connection reference"=w265:T1)  [unwired: 10 in, 1 out]
            n167 = case shown="\"清空历史\"" w268 {
              tunnel: w265 -> [w274 w318 w377 w420]
              tunnel: w267 -> [w279 w325 w384 _]
              tunnel: [w269 w317 w376 w420] -> w264
              tunnel: w266 -> [_ w312 w371 _]
              frame "清空历史" {
                w278 = 2  # 数据库表 名称列
                # "delete from 表，重新查询"
                n168 = property class="MCListbox (严格)"(reference=w279) -> ("ItemSyms"=w275:i32[], "Value"=w276:i32[], "ItemNames"=w277:string[][])  [unwired: 1 in, 2 out]
                n169 = Index Array(array=w277, index (col)=w278) -> (element=w273:string[])  [unwired: 1 in]
                n170 = for {
                  tunnel: w276 -> [w284] mode=indexing
                  tunnel: w275 -> [w288]
                  tunnel: w273 -> [w285]
                  shift-right: [w282] -> w270
                  shift-left: "清空累积单元历史记录：" -> [w283]
                  shift-right: [w281] -> w269
                  shift-left: w274 -> [w286]
                  w289 = 3  # 无记录
                  n171 = Index Array "项符号"(array=w288, index=w284) -> (element=w290:i32)
                  n172 = Not Equal?(x=w290, y=w289) -> (x != y?=w287:bool)
                  n173 = case shown="真" w287 {
                    tunnel: w286 -> [w291 w301]
                    tunnel: [w291 w300] -> w281
                    tunnel: w285 -> [_ w299]
                    tunnel: w284 -> [_ w298]
                    tunnel: w283 -> [w292 w296]
                    tunnel: [w292 w294] -> w282
                    frame False {
                      # "没有表，不执行"
                    }
                    frame True {
                      # "有记录的，可执行"
                      n174 = Index Array "探头名称"(array=w299, index=w298) -> (element=w295:string)
                      n175 = call <vilib>:"DB Tools Delete Data.vi"("condition"="", "table"=w295, "connection reference"=w301) -> ("error out"=w297:errorcluster, "connection reference out"=w300:T1)  [unwired: 7 in]
                      n176 = case shown="无错误" w297 {
                        tunnel: w296 -> [w305 w307]
                        tunnel: w295 -> [w304 _]
                        tunnel: [w303 w307] -> w294
                        frame No Error {
                          n177 = Concatenate Strings(w305, w304, "，" ("字符串")) -> (w303:string)
                        }
                        frame Error {
                          n178 = property on="信号-重连DB" class="Bool (严格)"("Val(Sgnl)"=FALSE ("值(信号)")) -> ()  [unwired: 2 in, 2 out]
                        }
                      }
                    }
                  }
                }
                n179 = flat-sequence {
                  tunnel: w269 -> [_]
                  frame #0 {
                    n180 = local read "查询条件"() -> (w280:T2)
                    n181 = property on="查询条件" class="Clust (严格)"("Val(Sgnl)"=w280) -> ()  [unwired: 2 in, 2 out]
                  }
                }
                n182 = call "状态栏-插入状态信息-35点监测专用.vi"("消息内容"=w270, "状态类型"=enum16{"全部", "报警", "通信", "设置"}."设置") -> ()  [unwired: 10 in]
              }
              frame "创建累积单元" {
                w320 = 1  # 探头名称列
                # "允许批量"
                n183 = property class="Arr (严格)"(reference=w312) -> (reference out=w310:refnum<vi>, "Value"=w311:T8)  [unwired: 1 in, 1 out]
                n184 = property class="MCListbox (严格)"(reference=w325) -> (reference out=w324:refnum<vi>, "ItemSyms"=w322:i32[], "Value"=w323:i32[], "ItemNames"=w321:string[][])  [unwired: 1 in, 1 out]
                n185 = Index Array(array=w321, index (col)=w320) -> (element=w319:string[])  [unwired: 1 in]
                n186 = for {
                  tunnel: w324 -> [_]
                  tunnel: w323 -> [w330] mode=indexing
                  tunnel: w322 -> [w341]
                  tunnel: w319 -> [w331]
                  tunnel: w318 -> [w337]
                  tunnel: [w336] -> w317
                  shift-right: [w334] -> w313
                  shift-left: w311 -> [w335]
                  shift-right: [w332] -> w314
                  shift-left: "创建累积单元：" -> [w333]
                  w338 = 3  # 无记录
                  # "判断并创建数据库表"
                  n187 = Index Array "项符号"(array=w341, index=w330) -> (element=w340:i32)
                  n188 = Index Array "探头名称"(array=w331, index=w330) -> (element=w329:string)
                  n189 = Equal?(x=w340, y=w338) -> (x = y?=w339:bool)
                  n190 = Empty String/Path?(string/path=w329) -> (empty?=w328:bool)
                  n191 = Not(x=w328) -> (.not. x?=w326:bool)
                  n192 = And(x=w339, y=w326) -> (x .and. y?=w327:bool)
                  n193 = case shown="真" w327 {
                    tunnel: w337 -> [w344 w352]
                    tunnel: [w344 w351] -> w336
                    tunnel: w335 -> [w343 w349]
                    tunnel: [w343 w348] -> w334
                    tunnel: w333 -> [w342 w347]
                    tunnel: [w342 w346] -> w332
                    tunnel: w329 -> [_ w345]
                    frame False {
                      # "不可创建"
                    }
                    frame True {
                      # "错误处理\n状态提示"
                      # "可创建"
                      n194 = call "添加设备.vi"("设备名称"=w345, "数据库连接引用 i"=w352) -> ("error out"=w350:errorcluster, "数据库连接引用 o"=w351:T1)  [unwired: 8 in]
                      n195 = case shown="无错误" w350 {
                        tunnel: w349 -> [w363 w366]
                        tunnel: w345 -> [w355 _]
                        tunnel: [w357 w366] -> w348
                        tunnel: w347 -> [w356 w365]
                        tunnel: [w353 w365] -> w346
                        frame No Error {
                          # "2mSv"
                          n196 = Get Date/Time In Seconds() -> (seconds since 1Jan1904=w360:timestamp)
                          n197 = Bundle By Name(cluster=T3 {"设备名称"="", "启用累积？"=FALSE, "起始时间"=timestamp(0 s since 1904-01-01), "累积剂量"=0.0, "累积报警阈值"=0.0} ("新元素/子数组"), "设备名称"=w355, "启用累积？"=TRUE, "起始时间"=w360, "累积报警阈值"=2000.0) -> (w358:T3)
                          n198 = Insert Into Array(array=w363, new element=w358) -> (w357:T8)  [unwired: 1 in]
                          n199 = Concatenate Strings(w356, w355, "，" ("字符串")) -> (w353:string)
                        }
                        frame Error {
                          n200 = property on="信号-重连DB" class="Bool (严格)"("Val(Sgnl)"=FALSE ("值(信号)")) -> ()  [unwired: 2 in, 2 out]
                        }
                      }
                    }
                  }
                }
                n201 = property class="Arr (严格)"(reference=w310, "Value"=w313) -> (error out=w308:errorcluster)  [unwired: 1 in, 1 out]
                n202 = property on="信号-刷新功能管理表" class="Bool (严格)"(error in=w308, "Val(Sgnl)"=FALSE ("值(信号)")) -> ()  [unwired: 1 in, 2 out]
                n203 = call "状态栏-插入状态信息-35点监测专用.vi"("消息内容"=w314, "状态类型"=enum16{"全部", "报警", "通信", "设置"}."设置") -> ()  [unwired: 10 in]
              }
              frame "删除累积单元" {
                w379 = 2  # 数据库表 名称列
                # "允许批量"
                n204 = property class="Arr (严格)"(reference=w371) -> (reference out=w369:refnum<vi>, "Value"=w370:T8)  [unwired: 1 in, 1 out]
                n205 = property class="MCListbox (严格)"(reference=w384) -> (reference out=w383:refnum<vi>, "ItemSyms"=w381:i32[], "Value"=w382:i32[], "ItemNames"=w380:string[][])  [unwired: 1 in, 1 out]
                n206 = Index Array(array=w380, index (col)=w379) -> (element=w378:string[])  [unwired: 1 in]
                n207 = for {
                  tunnel: w383 -> [_]
                  tunnel: w382 -> [w391] mode=indexing
                  tunnel: w381 -> [w396]
                  tunnel: w378 -> [w392]
                  tunnel: w377 -> [w390]
                  tunnel: [w389] -> w376
                  shift-right: [w387] -> w372
                  shift-left: w370 -> [w388]
                  shift-right: [w385] -> w373
                  shift-left: "删除累积单元：" -> [w386]
                  w393 = 3  # 无记录
                  # "判断并创建数据库表"
                  n208 = Index Array "项符号"(array=w396, index=w391) -> (element=w395:i32)
                  n209 = Not Equal?(x=w395, y=w393) -> (x != y?=w394:bool)
                  n210 = case shown="真" w394 {
                    tunnel: w392 -> [_ w409]
                    tunnel: w391 -> [_ w408]
                    tunnel: w390 -> [w399 w403]
                    tunnel: [w399 w402] -> w389
                    tunnel: w388 -> [w398 w407]
                    tunnel: [w398 w406] -> w387
                    tunnel: w386 -> [w397 w405]
                    tunnel: [w397 w404] -> w385
                    frame False {
                      # "不可删除"
                    }
                    frame True {
                      # "错误处理\n状态提示"
                      # "可删除"
                      n211 = Index Array "探头名称"(array=w409, index=w408) -> (element=w400:string)
                      n212 = call <vilib>:"DB Tools Drop Table.vi"("table"=w400, "connection reference"=w403) -> ("error out"=w401:errorcluster, "connection reference out"=w402:T1)  [unwired: 6 in]
                      n213 = case shown="无错误" w401 {
                        tunnel: w407 -> [w412 w419]
                        tunnel: w400 -> [w410 _]
                        tunnel: [w416 w419] -> w406
                        tunnel: w405 -> [w415 w418]
                        tunnel: [w413 w418] -> w404
                        frame No Error {
                          n214 = call "查找匹配累积剂量.vi"("探头名称"=w410, "累积剂量"=w412) -> ("匹配索引"=w411:i32)  [unwired: 7 in, 2 out]
                          n215 = Delete From Array(array=w412, index=w411) -> (array with subset deleted=w416:T8)  [unwired: 1 in, 1 out]
                          n216 = Concatenate Strings(w415, w410, "，" ("字符串")) -> (w413:string)
                        }
                        frame Error {
                          n217 = property on="信号-重连DB" class="Bool (严格)"("Val(Sgnl)"=FALSE ("值(信号)")) -> ()  [unwired: 2 in, 2 out]
                        }
                      }
                    }
                  }
                }
                n218 = property class="Arr (严格)"(reference=w369, "Value"=w372) -> (error out=w367:errorcluster)  [unwired: 1 in, 1 out]
                n219 = property on="信号-刷新功能管理表" class="Bool (严格)"(error in=w367, "Val(Sgnl)"=FALSE ("值(信号)")) -> ()  [unwired: 1 in, 2 out]
                n220 = call "状态栏-插入状态信息-35点监测专用.vi"("消息内容"=w373, "状态类型"=enum16{"全部", "报警", "通信", "设置"}."设置") -> ()  [unwired: 10 in]
              }
              frame "刷新", Default {
                # "从数据库刷新所有表名称  并 构建列表"
                n221 = property on="信号-刷新功能管理表" class="Bool (严格)"("Val(Sgnl)"=FALSE ("值(信号)")) -> ()  [unwired: 2 in, 2 out]
              }
            }
            n222 = call <vilib>:"DB Tools Close Connection.vi"("connection reference"=w264) -> ("error out"=w263:errorcluster)  [unwired: 6 in]
            n223 = call <vilib>:"Clear Errors.vi"("error in (no error)"=w263) -> ()  [unwired: 5 in, 2 out]
          }
          event "记录列表": Shortcut Menu Selection (User) {
            n224 = event-data() -> ("CtlRef"=w422:refnum<vi>, "ItemTag"=w423:string)  [unwired: 1 in, 6 out]
            n225 = case shown="\"导出文本文档\"" w423 {
              tunnel: w422 -> [w424 _]
              frame "复制", Default {
                # "已复制"
                n226 = call "复制文本-选中累积剂量.vi"("引用-数据列表"=w424) -> ()  [unwired: 9 in, 2 out]
              }
              frame "导出文本文档" {
                # "需生成 txt 文档"
                n227 = property on="信号-导出数据" class="Bool (严格)"("Val(Sgnl)"=FALSE ("值(信号)")) -> ()  [unwired: 2 in, 2 out]
              }
            }
          }
          event "记录列表": Mouse Up {
            w431 = -1  # 列首字符串
            # "列表内容排序"
            n228 = event-data() -> ("CtlRef"=w435:refnum<vi>, "Coords"=w434:T5)  [unwired: 1 in, 6 out]
            n229 = invoke class="多列列表框 (严格)" method="Point To Row Column"(reference=w435, "Point"=w434) -> ("CellPosition"=w433:T7)  [unwired: 5 in, 6 out]
            n230 = property class="多列列表框 (严格)" props=["ItemSyms", "Label", "Text", "ItemNames"](reference=w435) -> ("ItemSyms"=w427:i32[], "ItemNames"=w428:string[][])  [unwired: 1 in, 3 out]
            n231 = Unbundle By Name(w433) -> ("Row"=w432:i32, "Column"=w430:i32)
            n232 = local read "查询条件"() -> (w426:T2)
            n233 = Equal?(x=w431, y=w432) -> (x = y?=w429:bool)
            n234 = case shown="1" w430 {
              tunnel: w429 -> [w436 w451 _]
              tunnel: w428 -> [_ _ _]
              tunnel: w427 -> [_ _ _]
              tunnel: w426 -> [w437 w452 _]
              frame 1 {
                # "按 表名称 排序"
                n235 = case shown="真" w436 {
                  tunnel: w437 -> [_ w443]
                  frame False {
                  }
                  frame True {
                    # "点到列首"
                    n236 = Unbundle By Name(w443) -> ("优先排序"=w442:enum16{"表名优先", "记录时间优先"}, "排序方向"=w441:enum16{"升序", "降序"})
                    n237 = case shown="\"表名优先\", 默认" w442 {
                      selector: w442 -> [w444 _]
                      tunnel: w441 -> [w446 w450]
                      tunnel: [w445 w450] -> w440
                      tunnel: [w444 enum16{"表名优先", "记录时间优先"}."表名优先" ("优先排序")] -> w439
                      frame "表名优先", Default {
                        # "已是表名优先，\n则改变排序方向"
                        n238 = case shown="\"降序\"" w446 {
                          tunnel: [enum16{"升序", "降序"}."降序" ("排序方向") enum16{"升序", "降序"}."升序" ("排序方向")] -> w445
                          frame "升序", Default {
                          }
                          frame "降序" {
                          }
                        }
                      }
                      frame "记录时间优先" {
                        # "改为表名优先"
                      }
                    }
                    n239 = Bundle By Name(cluster=w443, "优先排序"=w439, "排序方向"=w440) -> (w438:T2)
                    n240 = property on="查询条件" class="Clust (严格)"("Val(Sgnl)"=w438) -> ()  [unwired: 2 in, 2 out]
                  }
                }
              }
              frame 2 {
                # "按 记录时间 排序"
                n241 = case shown="真" w451 {
                  tunnel: w452 -> [_ w458]
                  frame False {
                  }
                  frame True {
                    # "点在列首"
                    n242 = Unbundle By Name(w458) -> ("优先排序"=w457:enum16{"表名优先", "记录时间优先"}, "排序方向"=w456:enum16{"升序", "降序"})
                    n243 = case shown="\"记录时间优先\"" w457 {
                      selector: w457 -> [_ w461]
                      tunnel: w456 -> [w460 w463]
                      tunnel: [w460 w462] -> w455
                      tunnel: [enum16{"表名优先", "记录时间优先"}."记录时间优先" ("优先排序") w461] -> w454
                      frame "表名优先", Default {
                        # "改为时间优先"
                      }
                      frame "记录时间优先" {
                        # "已是时间优先，\n则改变排序方向"
                        n244 = case shown="\"降序\"" w463 {
                          tunnel: [enum16{"升序", "降序"}."降序" ("排序方向") enum16{"升序", "降序"}."升序" ("排序方向")] -> w462
                          frame "升序", Default {
                          }
                          frame "降序" {
                          }
                        }
                      }
                    }
                    n245 = Bundle By Name(cluster=w458, "优先排序"=w454, "排序方向"=w455) -> (w453:T2)
                    n246 = property on="查询条件" class="Clust (严格)"("Val(Sgnl)"=w453) -> ()  [unwired: 2 in, 2 out]
                  }
                }
              }
              frame 0, Default {
                # "其他列 未应用排序功能 不执行"
              }
            }
          }
          event "查询今日": Value Change {
            n247 = event-data() -> ("CtlRef"=w467:refnum<vi>, "NewVal"=w466:bool)  [unwired: 1 in, 4 out]
            n248 = case shown="真" w466 {
              tunnel: w467 -> [_ w469]
              frame False {
              }
              frame True {
                n249 = property class="Bool (严格)"(reference=w469, "Value"=FALSE ("值")) -> ()  [unwired: 1 in, 2 out]
                n250 = Get Date/Time In Seconds() -> (seconds since 1Jan1904=w477:timestamp)
                n251 = Seconds To Date/Time(time stamp (now)=w477) -> (date time rec=w476:T4)  [unwired: 1 in]
                n252 = Unbundle By Name(w476) -> ("年"=w475:i32, "月"=w474:i32, "日"=w473:i32)
                n253 = local write "起始年"(w475) -> ()
                n254 = local write "起始月"(w474) -> ()
                n255 = local write "起始日"(w473) -> ()
                n256 = local write "截止年"(w475) -> ()
                n257 = local write "截止月"(w474) -> ()
                n258 = local write "截止日"(w473) -> ()
                n259 = call "起始时间.vi"("起始日"=w473, "起始月"=w474, "起始年"=w475) -> ("起始时间"=w472:string)  [unwired: 8 in]
                n260 = call "截止时间.vi"("起始日"=w473, "起始月"=w474, "起始年"=w475) -> ("截止时间"=w471:string)  [unwired: 8 in]
                n261 = local read "查询条件"() -> (w478:T2)
                n262 = Bundle By Name(cluster=w478, "起始时间"=w472, "截止时间"=w471) -> (w470:T2)
                n263 = property on="查询条件" class="Clust (严格)"("Val(Sgnl)"=w470) -> ()  [unwired: 2 in, 2 out]
              }
            }
          }
          event "起始年", "起始月", "起始日", "截止年", "截止月", "截止日": Value Change {
            # "日期条件改变，查询"
            n264 = event-data() -> ()  [unwired: 1 in, 6 out]
            n265 = stacked-sequence {
              frame #0 {
                # "检测日期逻辑"
                n266 = local read "最小记录时间"() -> (w485:i32[])
                n267 = control-ref of="截止月"() -> (w480:refnum<vi>)
                n268 = control-ref of="截止年"() -> (w481:refnum<vi>)
                n269 = control-ref of="截止日"() -> (w479:refnum<vi>)
                n270 = control-ref of="起始月"() -> (w483:refnum<vi>)
                n271 = control-ref of="起始日"() -> (w482:refnum<vi>)
                n272 = control-ref of="起始年"() -> (w484:refnum<vi>)
                n273 = call "取值范围-年月日下拉取值范围.vi"("最小日期"=w485, "日"=w479, "月"=w480, "年"=w481) -> ()  [unwired: 7 in, 1 out]
                n274 = call "取值范围-年月日下拉取值范围.vi"("最小日期"=w485, "日"=w482, "月"=w483, "年"=w484) -> ()  [unwired: 7 in, 1 out]
              }
              frame #1 {
                # "赋值到查询条件"
                n275 = call "起始时间.vi"("起始日"="起始日", "起始月"="起始月", "起始年"="起始年") -> ("起始时间"=w491:string)  [unwired: 8 in]
                n276 = call "截止时间.vi"("起始日"="截止日", "起始月"="截止月", "起始年"="截止年") -> ("截止时间"=w492:string)  [unwired: 8 in]
                n277 = Less Or Equal?(x=w491, y=w492) -> (x <= y?=w489:bool)
                n278 = Select(t=w492, s=w489, f=w491) -> (s? t:f=w490:string)
                n279 = case shown="假" w489 {
                  tunnel: "起始年" -> [w500 _]
                  tunnel: "起始月" -> [w499 _]
                  tunnel: "起始日" -> [w498 _]
                  frame False {
                    # "逻辑异常，取最大值"
                    n280 = local write "截止年"(w500) -> ()
                    n281 = local write "截止月"(w499) -> ()
                    n282 = local write "截止日"(w498) -> ()
                  }
                  frame True {
                    # "逻辑正常"
                  }
                }
                n283 = local read "查询条件"() -> (w494:T2)
                n284 = Bundle By Name(cluster=w494, "起始时间"=w491, "截止时间"=w490) -> (w493:T2)
                n285 = property on="查询条件" class="Clust (严格)"("Val(Sgnl)"=w493) -> ()  [unwired: 2 in, 2 out]
              }
            }
          }
          event "从今天", "到今天": Value Change {
            w501 = "/" ("分隔符（/）")
            # "将起始日期 或 截止日期置为今日，不能冲突"
            n286 = event-data() -> ("CtlRef"=w520:refnum<vi>)  [unwired: 1 in, 5 out]
            n287 = property class="Bool"(reference=w520) -> ("Label.Text"=w519:string)  [unwired: 1 in, 2 out]
            n288 = Get Date/Time In Seconds() -> (seconds since 1Jan1904=w522:timestamp)
            n289 = Seconds To Date/Time(time stamp (now)=w522) -> (date time rec=w521:T4)  [unwired: 1 in]
            n290 = Equal?(x=w519, y="从今天") -> (x = y?=w512:bool)
            n291 = Unbundle By Name(w521) -> ("年"=w517:i32, "月"=w516:i32, "日"=w515:i32)
            n292 = case shown="真" w512 {
              tunnel: w517 -> [w527 w538]
              tunnel: w516 -> [w526 w537]
              tunnel: w515 -> [w525 w536]
              tunnel: [w523 w532] -> w513
              tunnel: [w524 w531] -> w503
              frame False {
                # "截止日期设为 “今日”"
                n293 = local read "起始年"() -> (w530:u16)
                n294 = local read "起始月"() -> (w528:u16)
                n295 = local read "起始日"() -> (w529:u16)
                n296 = call "截止时间.vi"("起始日"=w525, "起始月"=w526, "起始年"=w527) -> ("截止时间"=w523:string)  [unwired: 8 in]
                n297 = call "起始时间.vi"("起始日"=w529, "起始月"=w528, "起始年"=w530) -> ("起始时间"=w524:string)  [unwired: 8 in]
              }
              frame True {
                # "起始日期设为 “今日”"
                n298 = local read "截止年"() -> (w535:u16)
                n299 = local read "截止月"() -> (w534:u16)
                n300 = local read "截止日"() -> (w533:u16)
                n301 = call "起始时间.vi"("起始日"=w536, "起始月"=w537, "起始年"=w538) -> ("起始时间"=w531:string)  [unwired: 8 in]
                n302 = call "截止时间.vi"("起始日"=w533, "起始月"=w534, "起始年"=w535) -> ("截止时间"=w532:string)  [unwired: 8 in]
              }
            }
            n303 = Less Or Equal?(x=w503, y=w513) -> (x <= y?=w514:bool)
            n304 = Select(t=w513, s=w514, f=w503) -> (s? t:f=w502:string)
            n305 = call "转换-日期字符串至数值时间数组.vi"("分隔符（/）"=w501, "日期时间（或仅日期）字符串"=w502) -> ("D"=w506:i32, "M"=w507:i32, "Y"=w508:i32)  [unwired: 5 in, 2 out]
            n306 = call "转换-日期字符串至数值时间数组.vi"("分隔符（/）"=w501, "日期时间（或仅日期）字符串"=w503) -> ("D"=w509:i32, "M"=w510:i32, "Y"=w511:i32)  [unwired: 5 in, 2 out]
            n307 = local write "截止年"(w508) -> ()
            n308 = local write "截止月"(w507) -> ()
            n309 = local write "截止日"(w506) -> ()
            n310 = local write "起始年"(w511) -> ()
            n311 = local write "起始月"(w510) -> ()
            n312 = local write "起始日"(w509) -> ()
            n313 = local read "查询条件"() -> (w505:T2)
            n314 = Bundle By Name(cluster=w505, "起始时间"=w503, "截止时间"=w502) -> (w504:T2)
            n315 = property on="查询条件" class="Clust (严格)"("Val(Sgnl)"=w504) -> ()  [unwired: 2 in, 2 out]
          }
          event "查询条件": Value Change {
            # "查询数据库，获取结果并刷新数据列表"
            n316 = event-data() -> ("NewVal"=w541:T2)  [unwired: 1 in, 5 out]
            n317 = Unbundle By Name(w541) -> ("表名"=w540:string[])
            n318 = Empty Array?(array=w540) -> (empty?=w539:bool)
            n319 = case shown="假" w539 {
              tunnel: w541 -> [w546 _]
              frame False {
                # "有可查询的记录"
                n320 = call "连接数据库.vi"() -> ("error out"=w543:errorcluster, "connection reference"=w544:T1)  [unwired: 10 in]
                n321 = call "查询记录.vi"("错误输入"=w543, "查询条件"=w546, "数据库连接引用 i"=w544) -> ("error out"=w547:errorcluster, "查询结果"=w545:string[][], "数据库连接引用 o"=w542:T1)  [unwired: 6 in]
                n322 = call <vilib>:"DB Tools Close Connection.vi"("connection reference"=w542) -> ()  [unwired: 6 in, 1 out]
                n323 = case shown="无错误" w547 {
                  tunnel: w545 -> [w554 _]
                  frame No Error {
                    n324 = Array Size(array=w554) -> (size(s)=w553:i32[])
                    n325 = Index Array(array=w553) -> (element=w551:i32)  [unwired: 1 in]
                    n326 = call "今日-日期时间字符串.vi"() -> ("日期时间"=w552:string)  [unwired: 9 in, 2 out]
                    n327 = call "创建文本"("查询时间"=w552, "数目"=w551) -> ("Result"=w550:string)  [unwired: 12 in, 1 out]
                    n328 = local write "选中状态"("未选择数据" ("选中状态")) -> ()
                    n329 = local write "查询状态"(w550) -> ()
                  }
                  frame Error {
                    n330 = property on="信号-重连DB" class="Bool (严格)"("Val(Sgnl)"=FALSE ("值(信号)")) -> ()  [unwired: 2 in, 2 out]
                  }
                }
                n331 = property on="记录列表" class="MCListbox (严格)"("ItemNames"=w545, "Value"=i32[] [] ("记录列表")) -> ()  [unwired: 2 in, 2 out]
              }
              frame True {
                # "无可查询记录"
                n332 = property on="记录列表" class="MCListbox (严格)"("ItemNames"=string[][] [] ("项名"), "Value"=i32[] [] ("记录列表")) -> ()  [unwired: 2 in, 2 out]
                n333 = local write "查询状态"("未勾选任何设备" ("查询状态")) -> ()
                n334 = local write "选中状态"("未选则数据" ("查询状态")) -> ()
              }
            }
          }
          event "信号-刷新功能管理表": Value Change {
            n335 = event-data() -> ()  [unwired: 1 in, 6 out]
            n336 = call "连接数据库.vi"() -> ("error out"=w561:errorcluster, "connection reference"=w562:T1)  [unwired: 10 in]
            n337 = control-ref of="设备累积管理"() -> (w563:refnum<vi>)
            n338 = call "组件表-累积功能管理表.vi"("引用-累积功能管理列表"=w563, "error in (no error)"=w561, "DB 引用"=w562) -> ("error out"=w564:errorcluster, "数据库连接引用 o"=w560:T1)  [unwired: 6 in, 1 out]
            n339 = case shown="错误" w564 {
              tunnel: w563 -> [w565 _]
              frame No Error {
                n340 = call "从表中获取待查设备.vi"("引用-设备累积管理 i"=w565) -> ("选中的查询设备"=w567:string[])  [unwired: 10 in]
                n341 = local read "查询条件"() -> (w568:T2)
                n342 = Bundle By Name(cluster=w568, "表名"=w567) -> (w566:T2)
                n343 = local write "查询条件"(w566) -> ()
              }
              frame Error {
                n344 = property on="信号-重连DB" class="Bool (严格)"("Val(Sgnl)"=FALSE ("值(信号)")) -> ()  [unwired: 2 in, 2 out]
              }
            }
            n345 = call <vilib>:"DB Tools Close Connection.vi"("connection reference"=w560) -> ()  [unwired: 6 in, 1 out]
          }
          event "信号-重连DB": Value Change {
            # "重连数据库，并状态栏提示"
            n346 = event-data() -> ()  [unwired: 1 in, 6 out]
            n347 = stacked-sequence {
              tunnel: enum16{"全部", "报警", "通信", "设置"}."设置" ("状态类型") -> [w571 w574]
              frame #0 {
                # "提示重连 数据库"
                n348 = call "状态栏-插入状态信息-35点监测专用.vi"("消息内容"="出现错误，数据库操作过程异常，正在重连数据库……", "状态类型"=w571) -> ()  [unwired: 10 in]
              }
              frame #1 {
                # "重连数据库"
                n349 = call "连接数据库.vi"() -> ("error out"=w575:errorcluster, "connection reference"=w576:T1)  [unwired: 10 in]
                n350 = case shown="错误" w575 {
                  selector: w575 -> [_ w581]
                  tunnel: w576 -> [w577 _]
                  tunnel: w574 -> [_ _]
                  tunnel: ["数据库重连成功。" ("消息内容") w582] -> w573
                  frame No Error {
                    n351 = call <vilib>:"DB Tools Close Connection.vi"("connection reference"=w577) -> ()  [unwired: 6 in, 1 out]
                  }
                  frame Error {
                    w580 = "\r\n"
                    n352 = call "路径查找创建-报警记录清单.vi"() -> ("数据库路径"=w585:path)  [unwired: 8 in, 11 out]
                    n353 = Unbundle By Name(w581) -> ("source"=w579:string)
                    n354 = Path To String(path=w585) -> (string=w583:string)
                    n355 = Concatenate Strings("重连数据库失败，检查数据库文件是否存在" ("消息内容"), w580, w583, w580, w579) -> (w582:string)
                  }
                }
                n356 = call "状态栏-插入状态信息-35点监测专用.vi"("消息内容"=w573, "状态类型"=w574) -> ()  [unwired: 10 in]
              }
            }
          }
          event "信号-导出数据": Value Change {
            # "导出 txt 文件到目录，询问是否打开查看"
            n357 = event-data() -> ()  [unwired: 1 in, 6 out]
            n358 = control-ref of="记录列表"() -> (w588:refnum<vi>)
            n359 = call "复制文本-选中累积剂量.vi"("引用-数据列表"=w588) -> ("文本"=w587:string)  [unwired: 9 in, 1 out]
            n360 = Empty String/Path?(string/path=w587) -> (empty?=w586:bool)
            n361 = case shown="假" w586 {
              tunnel: w587 -> [w590 _]
              frame False {
                # "内容非空，可以写入文件"
                n362 = Get Date/Time In Seconds() -> (seconds since 1Jan1904=w598:timestamp)
                n363 = call "路径查找创建-报警记录清单.vi"() -> ("累积剂量导出目录"=w599:path)  [unwired: 8 in, 11 out]
                n364 = Format Date/Time String "导出时间_文件名"(time format string (%c)="%Y_%m_%d#%H_%M_%S.txt" ("时间格式字符串(%c)"), seconds (now)=w598) -> (date/time string=w589:string)  [unwired: 1 in]
                n365 = Build Path(base path=w599, name or relative path=w589) -> (appended path=w597:path)
                n366 = Write to Text File(file (use dialog)=w597, text=w590) -> (refnum out=w594:refnum<file>, cancelled=w596:bool, error out=w593:errorcluster)  [unwired: 2 in]
                n367 = Close File(refnum=w594, error in=w593) -> (path=w592:path, error out=w591:errorcluster)
                n368 = case shown="假" w596 {
                  tunnel: w589 -> [w605 _]
                  tunnel: w592 -> [w604 _]
                  tunnel: w591 -> [w602 _]
                  frame False {
                    # "已保存，提示"
                    n369 = call "显示对话框信息"("error in (no error)"=w602, "Message"=w605) -> ("error out"=w603:errorcluster, "打开"=w601:bool)  [unwired: 8 in]
                    n370 = case shown="真" w601 {
                      tunnel: w604 -> [_ w609]
                      tunnel: w603 -> [w606 w608]
                      tunnel: [w606 w607] -> w600
                      frame False {
                        # "不查看"
                      }
                      frame True {
                        # "立即查看"
                        n371 = call "cmd打开文件.vi"("error in (no error)"=w608, "文件路径"=w609) -> ("error out"=w607:errorcluster)  [unwired: 9 in]
                      }
                    }
                    n372 = call <vilib>:"Clear Errors.vi"("error in (no error)"=w600) -> ()  [unwired: 5 in, 2 out]
                  }
                  frame True {
                    # "取消"
                  }
                }
              }
              frame True {
                # "剪贴板空，不可写入文件，弹窗提示"
              }
            }
          }
          event "导出数据": Value Change {
            n373 = event-data() -> ()  [unwired: 1 in, 6 out]
            n374 = property on="信号-导出数据" class="Bool (严格)"("Val(Sgnl)"=FALSE ("值(信号)")) -> ()  [unwired: 2 in, 2 out]
          }
          event "查看导出目录": Value Change {
            # "打开目录"
            n375 = event-data() -> ()  [unwired: 1 in, 6 out]
            n376 = call "路径查找创建-报警记录清单.vi"() -> ("累积剂量导出目录"=w612:path)  [unwired: 8 in, 11 out]
            n377 = call "cmd打开文件夹.vi"("文件路径"=w612) -> ("error out"=w611:errorcluster)  [unwired: 10 in]
            n378 = call <vilib>:"Clear Errors.vi"("error in (no error)"=w611) -> ()  [unwired: 5 in, 2 out]
          }
        }
      }
      n379 = while {
        stop <- "停止？" stop-if-true
        w44 = 0 ("y")
        w42 = 10  # 5s
        # "滚动提示切换"
        n380 = feedback #1(w44) -> (w46:i32)
        n381 = Array Size(array="提示-设备列表[]") -> (size(s)=w38:i32)
        n382 = Array Size(array="提示-数据列表[]") -> (size(s)=w37:i32)
        n383 = Array Size(array="提示-条件区域[]") -> (size(s)=w39:i32)
        n384 = Greater Or Equal?(x=w46, y=w42) -> (x >= y?=w41:bool)
        n385 = Decrement(x=w38) -> (x-1=w36:i32)
        n386 = Select(t=w44, s=w41, f=w46) -> (s? t:f=w43:i32)
        n387 = Decrement(x=w37) -> (x-1=w34:i32)
        n388 = Decrement(x=w39) -> (x-1=w32:i32)
        n389 = Increment(x=w43) -> (x+1=w45:i32)
        n390 = feedback-in #1(w45) -> ()
        n391 = case shown="真" w41 {
          tunnel: w36 -> [_ w68]
          tunnel: w34 -> [_ w65]
          tunnel: "提示-数据列表[]" -> [_ w60]
          tunnel: "提示-设备列表[]" -> [_ w59]
          tunnel: w32 -> [_ w53]
          tunnel: "提示-条件区域[]" -> [_ w56]
          frame False {
            # "未到 5s"
          }
          frame True {
            w57 = 0 ("y")
            w58 = 0 ("y")
            w71 = 0 ("y")
            # "5s 到了"
            n392 = feedback #2(w71) -> (w70:i32)
            n393 = feedback #3(w58) -> (w66:i32)
            n394 = feedback #4(w57) -> (w52:i32)
            n395 = Greater?(x=w70, y=w68) -> (0:w69:bool)
            n396 = Greater?(x=w66, y=w65) -> (0:w67:bool)
            n397 = Greater?(x=w52, y=w53) -> (0:w51:bool)
            n398 = Select(t=w71, s=w69, f=w70) -> (s? t:f=w64:i32)
            n399 = Select(t=w58, s=w67, f=w66) -> (s? t:f=w61:i32)
            n400 = Select(t=w57, s=w51, f=w52) -> (s? t:f=w55:i32)
            n401 = Increment(x=w64) -> (x+1=w63:i32)
            n402 = feedback-in #2(w63) -> ()
            n403 = Increment(x=w61) -> (x+1=w62:i32)
            n404 = feedback-in #3(w62) -> ()
            n405 = Increment(x=w55) -> (x+1=w54:i32)
            n406 = feedback-in #4(w54) -> ()
            n407 = Index Array(array=w59, index=w64) -> (element=→"提示-设备列表":string)
            n408 = Index Array(array=w60, index=w61) -> (element=→"提示-数据列表":string)
            n409 = Index Array(array=w56, index=w55) -> (element=→"提示-条件区域":string)
          }
        }
        n410 = Wait (ms)(milliseconds to wait=u32 500 ("等待时间（毫秒）")) -> ()  [unwired: 1 out]
      }
    }
  }
